vi "GLdrv_FILE_TRANS_CLOSE.vi"(0 "Connection ID":T1, 11 "error in (no error)":errorcluster) -> (4 "Connection ID Out":T1, 15 "error out":errorcluster)   [LabVIEW 2017, in "GL860_Driver.lvlib"]
doc: "記録計本体内のファイルを転送します\nOPENでオープンしたファイルをクローズします\nファイルをOPENして転送がすべて終わった後は必ずCLOSEを送信\nしてクローズ処理を行ってください"
uses:
  GL860_Driver.lvlib
  ConnectionID.ctl
panel:
  out "Error Code":i16
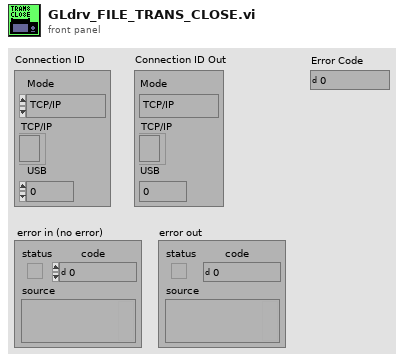
[diagram p1: front panel]
types:
  T1 = typedef "ConnectionID.ctl" = cluster{"Mode":enum16{"TCP/IP", "USB"}, "TCP/IP":refnum<k5>, "USB":i32}
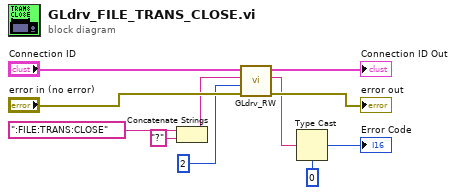
[diagram p0: block diagram]
diagram:
  n1 = Concatenate Strings(":FILE:TRANS:CLOSE" ("Command"), "?" ("string")) -> (w5:string)
  n2 = call "GLdrv_RW.vi"("error in (no error)"="error in (no error)", "Count(0:[CR+LF])"=u32 2, "data in"=w5, "Connection ID"="Connection ID") -> ("error out"=→"error out":errorcluster, "data out"=w1:string, "Connection ID Out"=→"Connection ID Out":T1)  [unwired: 3 in, 2 out]
  n3 = Type Cast(type=i16 0 ("Status"), x=w1) -> (*(type *) &x=→"Error Code":i16)
